vi "SPI.vi"() -> ()   [LabVIEW 2015]
uses:
  <vilib>/IEDriver/SPIandI2C/FPGA/Library/IP SPI&I2C.lvlib
  <vilib>/IEDriver/SPIandI2C/FPGA/Private/Initialize Port (SPI).vi
  <vilib>/IEDriver/SPIandI2C/FPGA/Private/IP Port (SPI).vi
  <vilib>/IEDriver/SPIandI2C/FPGA/Private/Configure Port (SPI).vi
  <vilib>/IEDriver/SPIandI2C/FPGA/Private/Write Port (SPI).vi
  <vilib>/IEDriver/SPIandI2C/FPGA/Private/Arm Port (SPI).vi
  <vilib>/IEDriver/SPIandI2C/FPGA/Private/Read Port (SPI).vi
panel:
  in  "SPI Protocol Action 0":T1(ring)=enum."Idle"
  out "SPI Protocol Output Data 0":u8
  in  "SPI Protocol Input Data 0":u8
  in  "SPI Protocol Configure 0":T2
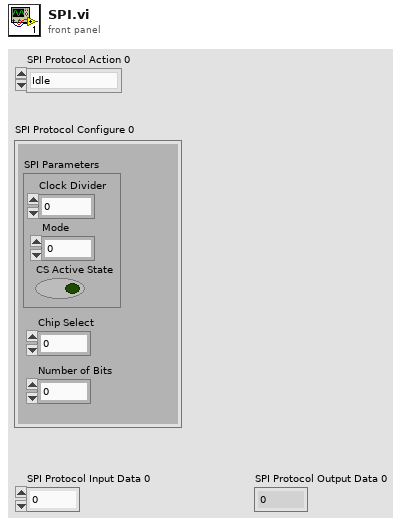
[diagram p1: front panel]
types:
  T1 = enum8{"Configure", "Write", "Arm", "Read", "Set Idle", "Idle"}
  T2 = cluster{"SPI Parameters":cluster{"Clock Divider":u32, "Mode":u8, "CS Active State":bool}, "Chip Select":u8, "Number of Bits":u16}
  T3 = cluster{"SCLK":refnum<k21>, "MISO":refnum<k21>, "MOSI":refnum<k21>, "CS 0":refnum<k21>}
  T4 = typedef "IP SPI&I2C.lvlib/Private Data (SPI).ctl" = cluster{"Arm Trigger":refnum<k21>, "API to IP Data":refnum<k21>, "IP to API Data":refnum<k21>, "Configure Register":refnum<k21>, "Configuration Lock":refnum<k21>}
  T5 = cluster{"Clock Divider":u32, "Mode":u8, "CS Active State":bool}
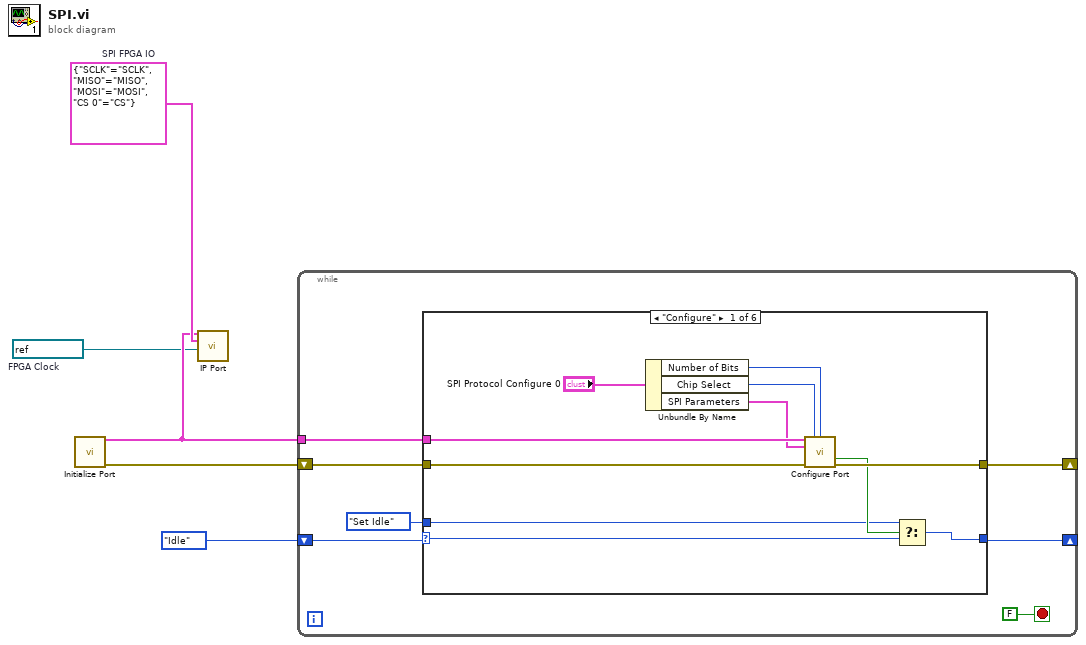
[diagram p0: block diagram]
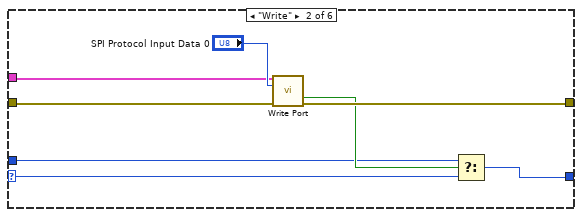
[diagram p2: hidden frame]
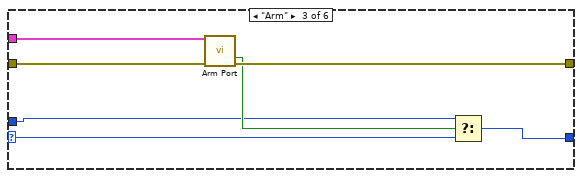
[diagram p3: hidden frame]
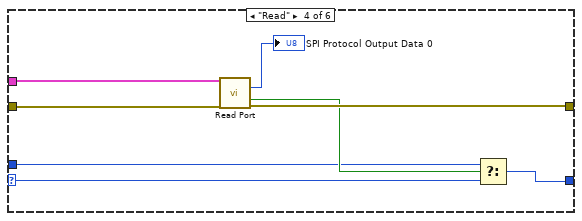
[diagram p4: hidden frame]
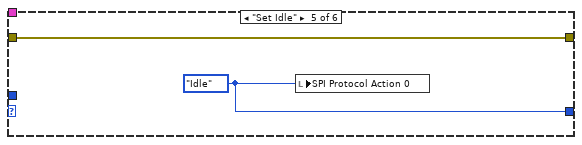
[diagram p5: hidden frame]
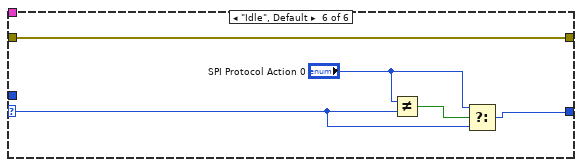
[diagram p6: hidden frame]
diagram:
  w5 = T3 {"SCLK"="SCLK", "MISO"="MISO", "MOSI"="MOSI", "CS 0"="CS"}  # SPI FPGA IO
  w1 = refnum<k21> "160MHz"  # FPGA Clock
  n1 = call-poly <vilib>:"Initialize Port.vi"() -> ("Private Data Out"=w2:T4, "error out"=w3:errorcluster)  [unwired: 14 in]
  n2 = call-poly <vilib>:"IP Port.vi"("Private Data In"=w2, "SPI FPGA IO"=w5, "FPGA Clock"=w1) -> ()  [unwired: 13 in]
  n3 = while {
    tunnel: w2 -> [w11]
    shift-right: [w9] -> _
    shift-left: w3 -> [w10]
    shift-right: [w7] -> _
    shift-left: T1."Idle" ("Action") -> [w8]
    stop <- FALSE stop-if-true
    n4 = case shown="\"Configure\"" w8 {
      selector: w8 -> [w14 w25 w33 w40 _ w50]
      tunnel: w11 -> [w23 w30 w38 w45 _ _]
      tunnel: w10 -> [w22 w29 w37 w44 w48 w53]
      tunnel: [w17 w28 w36 w43 w48 w53] -> w9
      tunnel: [w15 w27 w35 w42 w47 w51] -> w7
      tunnel: T1."Set Idle" ("Action") -> [w13 w24 w32 w39 _ _]
      frame "Configure" {
        n5 = Unbundle By Name("SPI Protocol Configure 0") -> ("Number of Bits"=w18:u16, "Chip Select"=w19:u8, "SPI Parameters"=w20:T5)
        n6 = call-poly <vilib>:"Configure Port.vi"("Private Data In"=w23, "Chip Select"=w19, "Number of Bits"=w18, "SPI Parameters"=w20, "error in"=w22) -> ("Done"=w16:bool, "error out"=w17:errorcluster)  [unwired: 8 in, 1 out]
        n7 = Select(t=w13, s=w16, f=w14) -> (s? t:f=w15:T1)
      }
      frame "Write" {
        n8 = call-poly <vilib>:"Write Port.vi"("Private Data In"=w30, "Data In"="SPI Protocol Input Data 0", "error in"=w29) -> ("Done"=w26:bool, "error out"=w28:errorcluster)  [unwired: 10 in, 1 out]
        n9 = Select(t=w24, s=w26, f=w25) -> (s? t:f=w27:T1)
      }
      frame "Arm" {
        n10 = call-poly <vilib>:"Arm Port.vi"("Private Data In"=w38, "error in"=w37) -> ("Done"=w34:bool, "error out"=w36:errorcluster)  [unwired: 11 in, 1 out]
        n11 = Select(t=w32, s=w34, f=w33) -> (s? t:f=w35:T1)
      }
      frame "Read" {
        n12 = call-poly <vilib>:"Read Port.vi"("Private Data In"=w45, "error in"=w44) -> ("Data Out"=→"SPI Protocol Output Data 0":u8, "Output Valid"=w41:bool, "error out"=w43:errorcluster)  [unwired: 10 in, 1 out]
        n13 = Select(t=w39, s=w41, f=w40) -> (s? t:f=w42:T1)
      }
      frame "Set Idle" {
        w47 = T1."Idle" ("Action")
        n14 = local write "SPI Protocol Action 0"(w47) -> ()
      }
      frame "Idle", Default {
        n15 = Not Equal?(x="SPI Protocol Action 0", y=w50) -> (x != y?=w52:bool)
        n16 = Select(t="SPI Protocol Action 0", s=w52, f=w50) -> (s? t:f=w51:T1)
      }
    }
  }
